vi "configure 8 or 12kHz 5 ch resonance PXI.vi"(6 "x resonant zoom voltage":dbl, 8 "error in":errorcluster, 9 "y-voltage":dbl=2.0, 10 "Start Delay (Ticks)":i16, 11 "lines (2pi) per frame":i32=100) -> (0 "error out":errorcluster, 1 "pixels per frame":dbl, 2 "FPGA VI Reference Out":refnum<k20>, 3 "AO task out":refnum<k21>, 4 "Actual Depth 3":u32)   [LabVIEW 2012]
uses:
  <vilib>/userdefined/High Color/nirio_resource_hc.ctl
  <vilib>/DAQmx/write.llb/DAQmx Write (Analog 2D DBL NChan NSamp).vi
  GFG/GFGbooleanGet.vi
  <vilib>/DAQmx/create/channels.llb/DAQmx Create Channel (AO-Voltage-Basic).vi
  <vilib>/DAQmx/configure/trigger.llb/DAQmx Start Trigger (Digital Edge).vi
  <vilib>/FPGAPlugInAG/PXIe-7962R/niLvFpga_Open_PXIe-7962R.vi
  <vilib>/FPGAPlugInAG/PXIe-7962R/niLvFpga_Abort_PXIe-7962R.vi
  <vilib>/Utility/error.llb/Error Cluster From Error Code.vi
  <vilib>/rvi/errors/niLvFpgaAdjustHostInterfaceError.vi
  <vilib>/FPGAPlugInAG/PXIe-7962R/niLvFpga_Run_PXIe-7962R.vi
  <vilib>/DAQmx/miscellaneous.llb/DAQmx Fill In Error Info.vi
  <vilib>/rvi/interface/nirviOpenFPGA/nirviOpenFPGA.xnode
  FPGA/current bitfiles/4chresonancescan_PXIe-7962R_5ch8or12kHzreson_gAN2W9JJOBI.lvbitx
  <vilib>/rvi/interface/nirviMethod/nirviMethod.xnode
  <vilib>/rvi/interface/nirviReadWriteControl/nirviReadWriteControl.xnode
  <vilib>/rvi/errors/niLvFpgaMergeErrorWithErrorCode.vi
  <vilib>/DAQmx/configure/timing.llb/DAQmx Timing (Sample Clock).vi
  GFG/GFG library.lvlib
  GFG/GFGnumericGet.vi
  GFG/GFGfpRefGet.vi
  <vilib>/FPGAPlugInAG/PXIe-7962R/niLvFpga_ConfigureFifo_PXIe-7962R.vi
  <vilib>/FPGAPlugInAG/PXIe-7962R/niLvFpga_ReadFifo_PXIe-7962R.vi
  <resource>/objmgr/daqmx.rc
  NiFpgaLv.dll
panel:
  in  "fpga input adapter sampling rate":i32=36000000
  in  "pockels.cell.ao.samples.per.s":dbl=1200000.0
  out "error out 2":errorcluster
  out "Actual Depth 2":u32
  out "Waveform Graph":dbl[][](graph)
  in  "Requested Depth":u32=100000000
  in  "RIO Device":T1="RIO0"
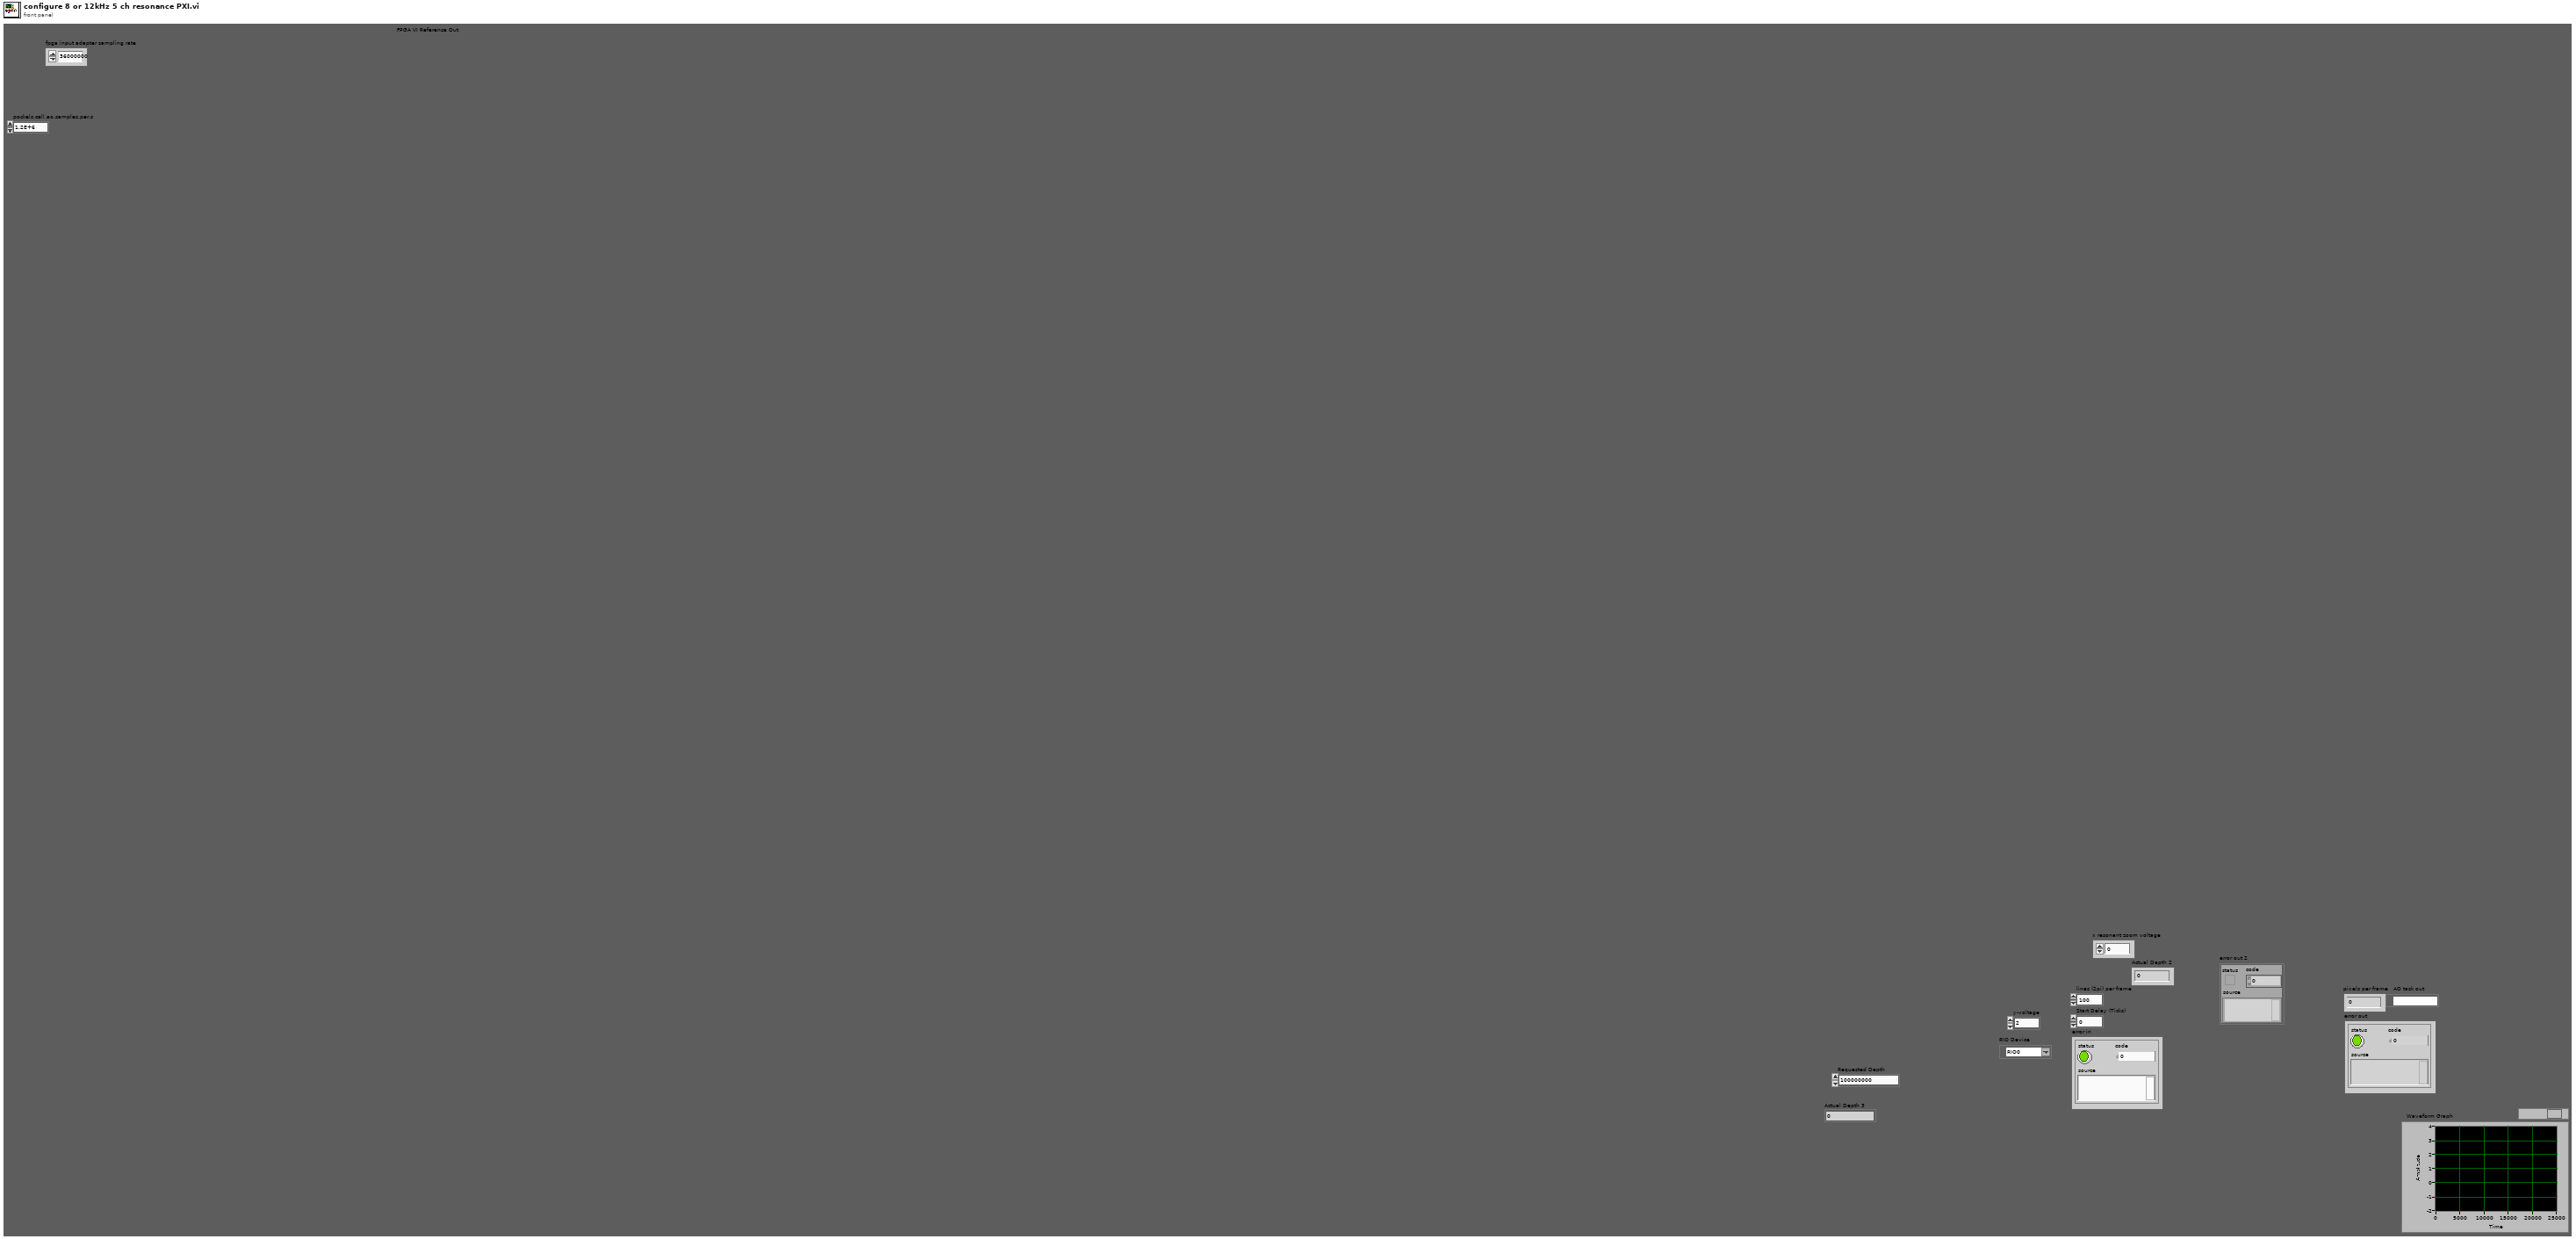
[diagram p1: front panel]
types:
  T1 = typedef "nirio_resource_hc.ctl" = tag
  T2 = enum8{"Enabled", "Disabled", "Disabled and Grayed Out"}
  T3 = cluster{"WaveformChartRef":refnum<vi>, "DigitalRef":refnum<vi>, "ArrayRef":refnum<vi>, "TabControlRef":refnum<vi>, "EnumRef":refnum<vi>, "RingRef":refnum<vi>, "BooleanRef":refnum<vi>, "KnobRef":refnum<vi>, "SlideRef":refnum<vi>, "PathRef":refnum<vi>, "StringRef":refnum<vi>, "ComboBox":refnum<vi>, "WaveformGraphRef":refnum<vi>}
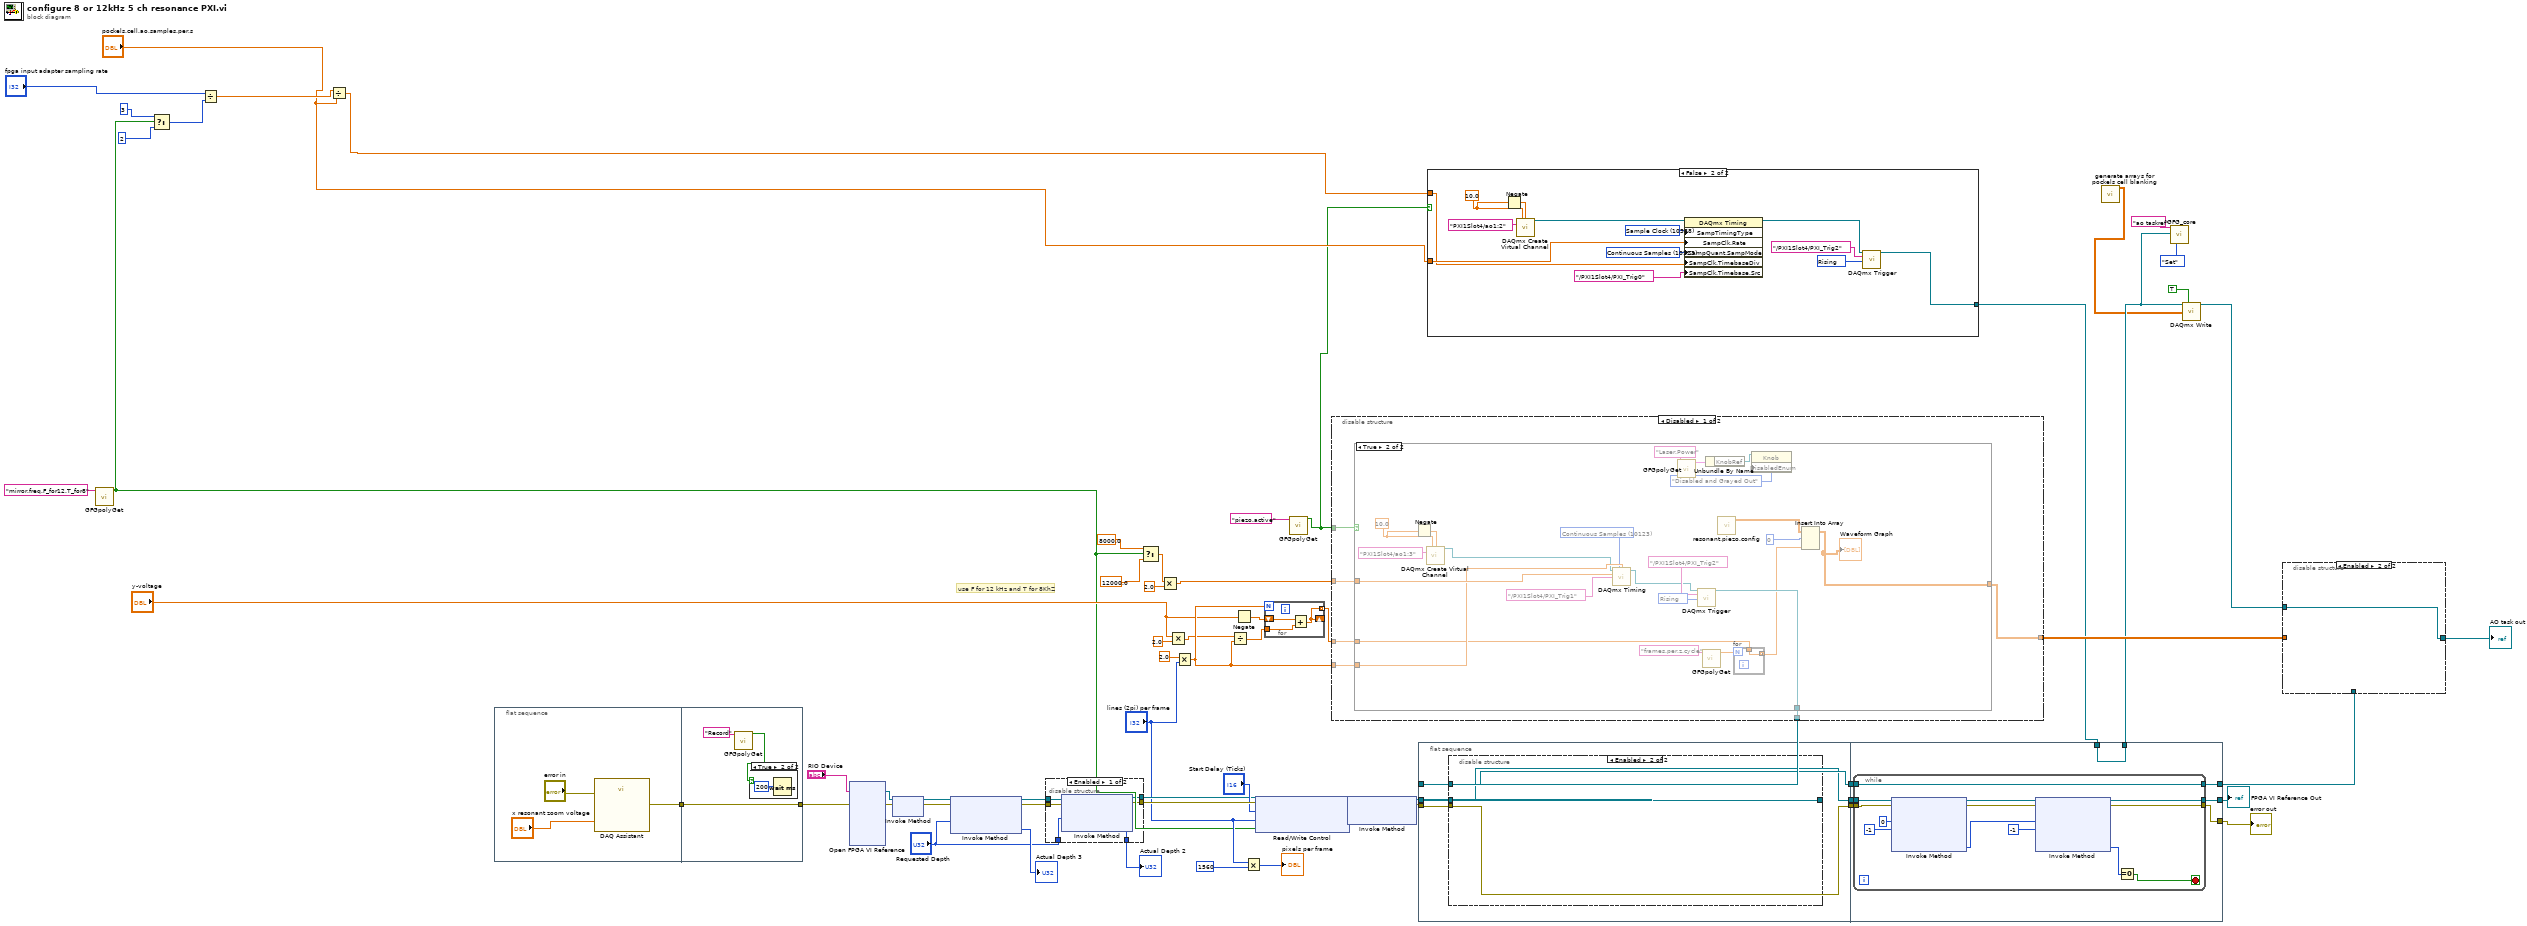
[diagram p0: block diagram]
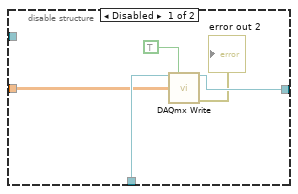
[diagram p2: hidden frame]
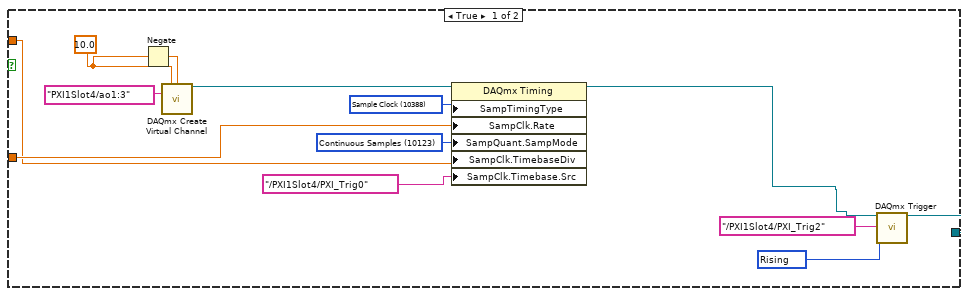
[diagram p3: hidden frame]
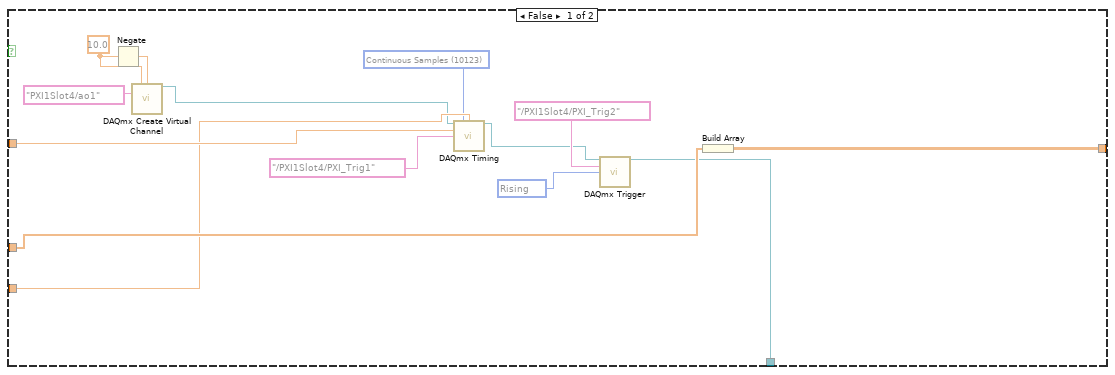
[diagram p4: hidden frame]
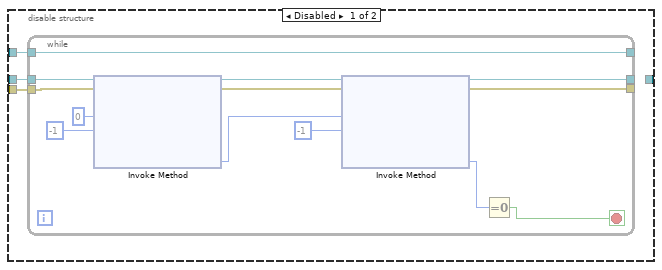
[diagram p7: hidden frame]
diagram:
  # "use F for 12 kHz and T for 8KhZ"
  n1 = call-poly "GFGpolyGet.vi"("Variable Name in"="mirror.freq.F_for12.T_for8") -> ("Boolean"=w9:bool)  [unwired: 10 in]
  n2 = Select(t=3, s=w9, f=2) -> (s? t:f=w15:i32)
  n3 = Divide(x="fpga input adapter sampling rate", y=w15) -> (x/y=w13:dbl)
  n4 = Divide(x=w13, y="pockels.cell.ao.samples.per.s") -> (x/y=w11:dbl)
  n5 = flat-sequence {
    tunnel: [w63] -> w33
    tunnel: [w68] -> w40
    tunnel: w33 -> [w68]
    frame #0 {
      n6 = call "DAQ Assistant"("data"="x resonant zoom voltage", "error in"="error in") -> ("error out"=w63:errorcluster)  [unwired: 16 in, 1 out]
    }
    frame #1 {
      n7 = call-poly "GFGpolyGet.vi"("Variable Name in"="Record") -> ("Boolean"=w66:bool)  [unwired: 10 in]
      n8 = case shown="True" w66 {
        frame False {
        }
        frame True {
          n9 = Wait (ms)(milliseconds to wait=u32 200) -> ()  [unwired: 1 out]
        }
      }
    }
  }
  n10 = xnode "Open FPGA VI Reference"("error in"=w40, "resource name"="RIO Device") -> ("FPGA VI Reference Out"=w60:refnum<k20>, "error out"=w61:errorcluster)
  n11 = xnode "Invoke Method"("FPGA VI Reference In"=w60, "error in"=w61) -> ("FPGA VI Reference Out"=w26:refnum<k20>, "error out"=w27:errorcluster)
  n12 = xnode "Invoke Method"("FPGA VI Reference In"=w26, "error in"=w27, "Requested Depth"="Requested Depth") -> ("FPGA VI Reference Out"=w36:refnum<k20>, "error out"=w35:errorcluster, "Actual Depth"=→"Actual Depth 3":u32)
  n13 = disable-structure shown="Enabled" {
    disable-tunnel: [w75 w76] -> w57
    disable-tunnel: w36 -> [w74 w77]
    disable-tunnel: w35 -> [w73 w76]
    disable-tunnel: [w72 _] -> w32
    disable-tunnel: "Requested Depth" -> [w71 _]
    disable-tunnel: [w70 w77] -> w30
    frame Enabled {
      n14 = xnode "Invoke Method"("FPGA VI Reference In"=w74, "error in"=w73, "Requested Depth"=w71) -> ("FPGA VI Reference Out"=w70:refnum<k20>, "error out"=w75:errorcluster, "Actual Depth"=w72:u32)
    }
    frame Disabled {
    }
  }
  "Actual Depth 2" <- w32
  n15 = Select(t=8000.0 ("rate"), s=w9, f=12000.0 ("rate")) -> (s? t:f=w23:dbl)
  n16 = Multiply(x=w23, y=2.0) -> (x*y=w50:dbl)
  n17 = Multiply(x="y-voltage", y=2.0) -> (x*y=w45:dbl)
  n18 = Multiply(x=2.0, y="lines (2pi) per frame") -> (x*y=w49:dbl)
  n19 = Divide(x=w45, y=w49) -> (x/y=w43:dbl)
  n20 = Negate(x="y-voltage") -> (-x=w44:dbl)
  n21 = Multiply(x="lines (2pi) per frame", y=i16 1560 ("samples per period")) -> (x*y=→"pixels per frame":i32)
  n22 = xnode "Read/Write Control"("FPGA VI Reference In"=w30, "error in"=w57, "Start Delay (Ticks)"="Start Delay (Ticks)", "lines at once"="lines (2pi) per frame", "frequency (T:8kHz F:12kHz)"=w9) -> ("FPGA VI Reference Out"=w59:refnum<k20>, "error out"=w58:errorcluster)
  n23 = for {
    N: w49 -> [_]
    tunnel: w43 -> [w79]
    shift-right: [w78] -> _
    shift-left: w44 -> [w80]
    tunnel: [w78] -> w52 mode=indexing
    n24 = Add(x=w80, y=w79) -> (x+y=w78:dbl)
  }
  n25 = call-poly "GFGpolyGet.vi"("Variable Name in"="piezo.active") -> ("Boolean"=w8:bool)  [unwired: 10 in]
  n26 = disable-structure shown="Disabled" {
    disable-tunnel: w52 -> [w86 _]
    disable-tunnel: w50 -> [w85 _]
    disable-tunnel: w49 -> [w84 _]
    disable-tunnel: [w83 _] -> w42
    disable-tunnel: [w82 _] -> w39
    disable-tunnel: w8 -> [w81 _]
    frame Disabled {
      n27 = case shown="True" w81 {
        tunnel: w86 -> [w100 w107]
        tunnel: w85 -> [w98 w122]
        tunnel: w84 -> [w95 w119]
        tunnel: [w89 w113] -> w83
        tunnel: [w87 w109] -> w82
        frame False {
          w99 = 10280 items=["Rising"=10280, "Falling"=10171] ("edge")
          w92 = 10123 items=["Finite Samples"=10178, "Continuous Samples"=10123, "Hardware Timed Single Point"=12522] ("sample mode")
          w93 = 10.0 ("maximum value")
          n28 = Negate(x=w93) -> (-x=w94:dbl)
          n29 = call-poly <vilib>:"DAQmx Create Virtual Channel.vi"("maximum value"=w93, "minimum value"=w94, "physical channels"=tag "PXI1Slot4/ao1") -> ("task out"=w90:refnum<k21>)  [unwired: 11 in, 1 out]
          n30 = call-poly <vilib>:"DAQmx Timing.vi"("task/channels in"=w90, "sample mode"=w92, "samples per channel"=w95, "rate"=w98, "source"=tag "/PXI1Slot4/PXI_Trig1") -> ("task out"=w88:refnum<k21>)  [unwired: 9 in, 1 out]
          n31 = call-poly <vilib>:"DAQmx Trigger.vi"("task/channels in"=w88, "source"=tag "/PXI1Slot4/PXI_Trig2", "edge"=w99) -> ("task out"=w89:refnum<k21>)  [unwired: 11 in, 1 out]
          n32 = Build Array(w100) -> (w87:dbl[][])
        }
        frame True {
          w123 = 10280 items=["Rising"=10280, "Falling"=10171] ("edge")
          w116 = 10123 items=["Finite Samples"=10178, "Continuous Samples"=10123, "Hardware Timed Single Point"=12522] ("sample mode")
          w117 = 10.0 ("maximum value")
          n33 = Negate(x=w117) -> (-x=w118:dbl)
          n34 = call-poly <vilib>:"DAQmx Create Virtual Channel.vi"("maximum value"=w117, "minimum value"=w118, "physical channels"=tag "PXI1Slot4/ao1:3") -> ("task out"=w114:refnum<k21>)  [unwired: 11 in, 1 out]
          n35 = call-poly <vilib>:"DAQmx Timing.vi"("task/channels in"=w114, "sample mode"=w116, "samples per channel"=w119, "rate"=w122, "source"=tag "/PXI1Slot4/PXI_Trig1") -> ("task out"=w112:refnum<k21>)  [unwired: 9 in, 1 out]
          n36 = call-poly "GFGpolyGet.vi"("Variable Name in"="Laser.Power") -> ("output cluster"=w104:T3)  [unwired: 9 in, 1 out]
          n37 = call-poly <vilib>:"DAQmx Trigger.vi"("task/channels in"=w112, "source"=tag "/PXI1Slot4/PXI_Trig2", "edge"=w123) -> ("task out"=w113:refnum<k21>)  [unwired: 11 in, 1 out]
          n38 = call-poly "GFGpolyGet.vi"("Variable Name in"="frames.per.z.cycle" ("Tag in")) -> ("Numeric"=w106:dbl)  [unwired: 9 in, 1 out]
          n39 = Unbundle By Name(w104) -> ("KnobRef"=w101:refnum<vi>)
          n40 = call "resonant.piezo.config.vi"() -> ("appended array"=w111:dbl[][])  [unwired: 11 in]
          n41 = for {
            N: w106 -> [_]
            tunnel: w107 -> [w124]
            tunnel: [w124] -> w105 mode=concatenating
          }
          n42 = property class="Knob"(reference=w101, "DisabledEnum"=T2."Disabled and Grayed Out" ("Disabled")) -> ()  [unwired: 1 in, 2 out]
          n43 = Insert Into Array(array=w111, index (row)=0 ("disabled index (col)"), new element=w105) -> (w109:dbl[][])  [unwired: 1 in]
          "Waveform Graph" <- w109
        }
      }
    }
    frame Enabled {
    }
  }
  n44 = xnode "Invoke Method"("FPGA VI Reference In"=w59, "error in"=w58) -> ("FPGA VI Reference Out"=w54:refnum<k20>, "error out"=w53:errorcluster)  [unwired: 1 in]
  n45 = flat-sequence {
    tunnel: w54 -> [w125]
    tunnel: [w125] -> w22
    tunnel: w53 -> [w127]
    tunnel: [w127] -> w21
    tunnel: w42 -> [w126]
    tunnel: [w126] -> w20
    tunnel: w22 -> [w151]
    tunnel: w21 -> [w150]
    tunnel: w20 -> [w149]
    tunnel: [w148] -> w41
    tunnel: [w146] -> w34
    tunnel: [w147] -> w1
    tunnel: w7 -> [w145]
    tunnel: [w145] -> w4
    frame #0 {
      n46 = disable-structure shown="Enabled" {
        disable-tunnel: w125 -> [w130 w144]
        disable-tunnel: w127 -> [w129 _]
        disable-tunnel: w126 -> [w128 _]
        disable-tunnel: [_ w144] -> _
        frame Disabled {
          n47 = while {
            tunnel: w130 -> [w143]
            tunnel: w129 -> [w137]
            tunnel: [w135] -> _
            tunnel: [w134] -> _
            tunnel: w128 -> [w133]
            tunnel: [w133] -> _
            stop <- w138 stop-if-true
            n48 = xnode "Invoke Method"("FPGA VI Reference In"=w143, "error in"=w137, "Number of Elements"=u32 0, "Timeout (ms)"=-1) -> ("FPGA VI Reference Out"=w139:refnum<k20>, "error out"=w136:errorcluster, "Elements Remaining"=w132:u32)  [unwired: 1 out]
            n49 = xnode "Invoke Method"("FPGA VI Reference In"=w139, "error in"=w136, "Number of Elements"=w132, "Timeout (ms)"=-1) -> ("FPGA VI Reference Out"=w135:refnum<k20>, "error out"=w134:errorcluster, "Elements Remaining"=w131:u32)  [unwired: 1 out]
            n50 = Equal To 0?(x=w131) -> (x = 0?=w138:bool)
          }
        }
        frame Enabled {
        }
      }
    }
    frame #1 {
      n51 = while {
        tunnel: w151 -> [w164]
        tunnel: w150 -> [w156]
        tunnel: [w154] -> w147
        tunnel: [w153] -> w146
        tunnel: w149 -> [w152]
        tunnel: [w152] -> w148
        stop <- w157 stop-if-true
        n52 = xnode "Invoke Method"("FPGA VI Reference In"=w164, "error in"=w156, "Number of Elements"=u32 0, "Timeout (ms)"=-1) -> ("FPGA VI Reference Out"=w160:refnum<k20>, "error out"=w155:errorcluster, "Elements Remaining"=w159:u32)  [unwired: 1 out]
        n53 = xnode "Invoke Method"("FPGA VI Reference In"=w160, "error in"=w155, "Number of Elements"=w159, "Timeout (ms)"=-1) -> ("FPGA VI Reference Out"=w154:refnum<k20>, "error out"=w153:errorcluster, "Elements Remaining"=w158:u32)  [unwired: 1 out]
        n54 = Equal To 0?(x=w158) -> (x = 0?=w157:bool)
      }
    }
  }
  n55 = case shown="False" w8 {
    tunnel: "pockels.cell.ao.samples.per.s" -> [w170 w183]
    tunnel: [w165 w180] -> w7
    tunnel: w11 -> [w169 w182]
    frame True {
      w168 = 10280 items=["Rising"=10280, "Falling"=10171] ("edge")
      w173 = 10388 items=["Sample Clock"=10388, "Burst Handshake"=12548, "Handshake"=10389, "Implicit"=10451, "On Demand"=10390, "Change Detection"=12504, "Pipelined Sample Clock"=14668] ("SampTimingType")
      w174 = 10123 items=["Finite Samples"=10178, "Continuous Samples"=10123, "Hardware Timed Single Point"=12522] ("SampQuant.SampMode")
      w176 = 10.0 ("maximum value")
      n56 = Negate(x=w176) -> (-x=w177:dbl)
      n57 = call-poly <vilib>:"DAQmx Create Virtual Channel.vi"("maximum value"=w176, "minimum value"=w177, "physical channels"=tag "PXI1Slot4/ao1:3") -> ("task out"=w171:refnum<k21>)  [unwired: 11 in, 1 out]
      n58 = property class="DAQmx Timing"(reference=w171, "SampTimingType"=w173, "SampClk.Rate"=w170, "SampQuant.SampMode"=w174, "SampClk.TimebaseDiv"=w169, "SampClk.Timebase.Src"=tag "/PXI1Slot4/PXI_Trig0" ("SampClk.Src")) -> (reference out=w166:refnum<k21>)  [unwired: 1 in, 1 out]
      n59 = call-poly <vilib>:"DAQmx Trigger.vi"("task/channels in"=w166, "source"=tag "/PXI1Slot4/PXI_Trig2", "edge"=w168) -> ("task out"=w165:refnum<k21>)  [unwired: 11 in, 1 out]
    }
    frame False {
      w179 = 10280 items=["Rising"=10280, "Falling"=10171] ("edge")
      w186 = 10388 items=["Sample Clock"=10388, "Burst Handshake"=12548, "Handshake"=10389, "Implicit"=10451, "On Demand"=10390, "Change Detection"=12504, "Pipelined Sample Clock"=14668] ("SampTimingType")
      w187 = 10123 items=["Finite Samples"=10178, "Continuous Samples"=10123, "Hardware Timed Single Point"=12522] ("SampQuant.SampMode")
      w189 = 10.0 ("maximum value")
      n60 = Negate(x=w189) -> (-x=w190:dbl)
      n61 = call-poly <vilib>:"DAQmx Create Virtual Channel.vi"("maximum value"=w189, "minimum value"=w190, "physical channels"=tag "PXI1Slot4/ao1:2") -> ("task out"=w184:refnum<k21>)  [unwired: 11 in, 1 out]
      n62 = property class="DAQmx Timing"(reference=w184, "SampTimingType"=w186, "SampClk.Rate"=w183, "SampQuant.SampMode"=w187, "SampClk.TimebaseDiv"=w182, "SampClk.Timebase.Src"=tag "/PXI1Slot4/PXI_Trig0" ("SampClk.Src")) -> (reference out=w181:refnum<k21>)  [unwired: 1 in, 1 out]
      n63 = call-poly <vilib>:"DAQmx Trigger.vi"("task/channels in"=w181, "source"=tag "/PXI1Slot4/PXI_Trig2", "edge"=w179) -> ("task out"=w180:refnum<k21>)  [unwired: 11 in, 1 out]
    }
  }
  n64 = call "generate arrays for pockels cell blanking.vi"() -> ("Array"=w2:dbl[][])  [unwired: 11 in]
  n65 = call "GFG_core.vi"("Variable Name in"="ao taskref", "Variant in"=w4, "Action"=enum16{"Init", "Set", "Get"}."Set") -> ()  [unwired: 10 in, 7 out]
  n66 = call-poly <vilib>:"DAQmx Write.vi"("task/channels in"=w4, "auto start"=TRUE, "data"=w2) -> ("task out"=w6:refnum<k21>)  [unwired: 10 in, 2 out]
  n67 = disable-structure shown="Enabled" {
    disable-tunnel: [w195 w196] -> w51
    disable-tunnel: w41 -> [w193 _]
    disable-tunnel: w39 -> [w192 _]
    disable-tunnel: w6 -> [_ w196]
    frame Disabled {
      n68 = call-poly <vilib>:"DAQmx Write.vi"("task/channels in"=w193, "auto start"=TRUE, "data"=w192) -> ("task out"=w195:refnum<k21>, "error out"=→"error out 2":errorcluster)  [unwired: 10 in, 1 out]
    }
    frame Enabled {
    }
  }
  "AO task out" <- w51
  "error out" <- w34
  "FPGA VI Reference Out" <- w1
